vi "SubVIs abbrechen.vi"(6 "Aktionen":enum16{"Setzen", "abbrechen"}(ring), 8 "error in":errorcluster caption="error out", 11 "vi referenzen":refnum<vi>[](array[refnum])) -> ()   [LabVIEW 2020, in "allgemeine Sub-VIs.lvlib"]
uses:
  allgemeine Sub-VIs.lvlib
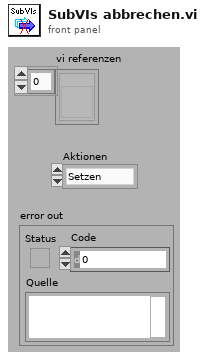
[diagram p1: front panel]
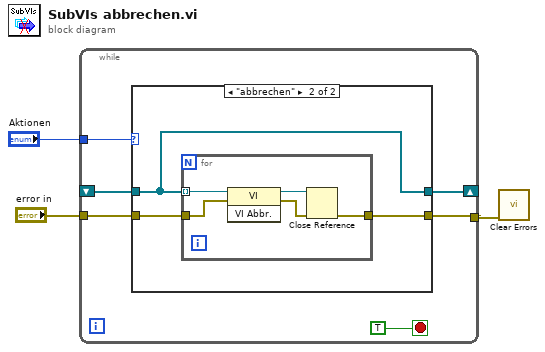
[diagram p0: block diagram]
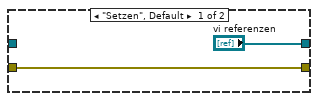
[diagram p2: hidden frame]
diagram:
  n1 = while {
    tunnel: [w8] -> w1
    tunnel: "error in" -> [w7]
    tunnel: "Aktionen" -> [w6]
    shift-right: [w5] -> _
    shift-left: _ -> [w4]
    stop <- TRUE stop-if-true
    n2 = case shown="\"abbrechen\"" w6 {
      tunnel: [w10 w14] -> w8
      tunnel: w7 -> [w10 w13]
      tunnel: ["vi referenzen" w12] -> w5
      tunnel: w4 -> [_ w12]
      frame "Setzen", Default {
      }
      frame "abbrechen" {
        n3 = for {
          tunnel: w12 -> [w16] mode=indexing
          tunnel: w13 -> [w15]
          tunnel: [w19] -> w14
          n4 = invoke class="VI" method="VI Abbr."(reference=w16, error in=w15) -> (reference out=w17:refnum<vi>, error out=w18:errorcluster)  [unwired: 1 in, 1 out]
          n5 = Close Reference(reference=w17, error in (no error)=w18) -> (error out=w19:errorcluster)
        }
      }
    }
  }
  n6 = call <vilib>:"Clear Errors.vi"("error in (no error)"=w1) -> ()  [unwired: 1 in, 6 out]
